vi "Test Gmail Auth.vi"() -> ()   [LabVIEW 2020]
uses:
  Gmail API/Mail Address.ctl
  Gmail API/Gmail/Gmail.lvclass
  <vilib>/IlluminatedG/IG OAuth2/OAuth2/Google/Google.lvclass
  C:/Program Files (x86)/National Instruments/LabVIEW 2020/vi.lib/IlluminatedG/IG OAuth2/OAuth2/OAuth2/OAuth2.lvclass
  <vilib>/IlluminatedG/IG OAuth2/OAuth2/OAuth2/Set Scopes.vi
  <vilib>/IlluminatedG/IG OAuth2/OAuth2/OAuth2/Launch Async Auth.vi
  Gmail API/Gmail/Add To.vi
  Gmail API/Gmail/Set Subject.vi
  Gmail API/Gmail/Set Content-Type.vi
  Gmail API/Gmail/Set Body.vi
  <vilib>/IlluminatedG/IG HTTP Utils/HTTP Utils/Response/Response.lvclass
  <vilib>/IlluminatedG/IG OAuth2/OAuth2/Authorization/Authorization.lvclass
  <vilib>/IlluminatedG/IG OAuth2/OAuth2/Client/Client.lvclass
  <vilib>/IlluminatedG/IG OAuth2/OAuth2/OAuth2/OAuth2.lvclass
  <vilib>/IlluminatedG/IG OAuth2/OAuth2/Async Authorization/Async Authorization.lvclass
  Gmail API/Gmail API.lvlib
panel:
  in  "Name":string
  in  "Content-Type":string
  in  "Body":string
  in  "Subject":string
  in  "Email":string
  in  "From Account (Prompt)":string
  in  "Secret":string
  in  "ID":string
  out "error out":errorcluster
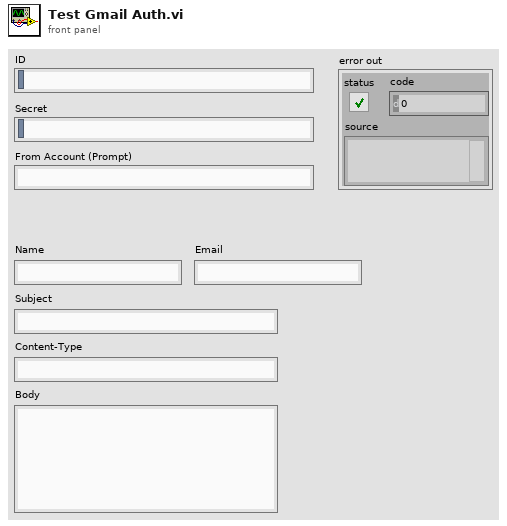
[diagram p1: front panel]
types:
  T1 = typedef "Gmail API.lvlib/Mail Address.ctl" = cluster{"Name":string, "Email":string}
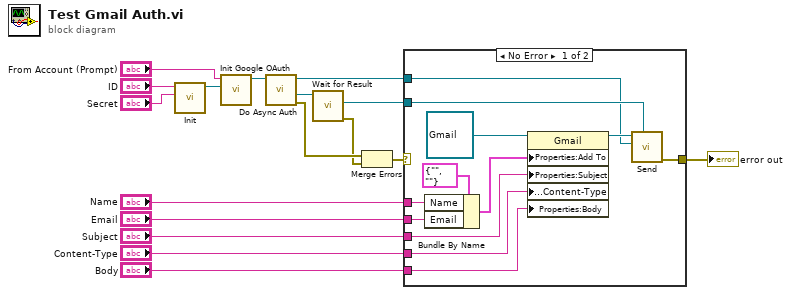
[diagram p0: block diagram]
diagram:
  n1 = call <vilib>:"Init.vi"("Secret"="Secret", "ID"="ID") -> ("Client out"=w2:refnum<class "Client.lvclass">)  [unwired: 9 in]
  n2 = call <vilib>:"Init Google OAuth.vi"("OAuth2:Client"=w2, "Account (Prompt)"="From Account (Prompt)") -> ("Google out"=w3:refnum<class "Google.lvclass">)  [unwired: 8 in, 1 out]
  n3 = call <vilib>:"Do Async Auth.vi"("OAuth2 in"=w3) -> ("error out"=w14:errorcluster, "Async Authentication"=w15:refnum<class "Async Authorization.lvclass">, "OAuth2 out"=w10:refnum<class "Google.lvclass">)  [unwired: 8 in]
  n4 = call <vilib>:"Wait for Result.vi"("Async Authorization in"=w15) -> ("error out"=w13:errorcluster, "Authorization"=w11:refnum<class "Authorization.lvclass">)  [unwired: 8 in, 1 out]
  n5 = Merge Errors(w14, w13) -> (w12:errorcluster)
  n6 = case shown="No Error" w12 {
    selector: w12 -> [_ w30]
    tunnel: w11 -> [w20 _]
    tunnel: w10 -> [w19 _]
    tunnel: "Email" -> [w27 _]
    tunnel: "Subject" -> [w25 _]
    tunnel: "Content-Type" -> [w24 _]
    tunnel: "Body" -> [w23 _]
    tunnel: "Name" -> [w28 _]
    tunnel: [w18 w30] -> w4
    frame No Error {
      n7 = Bundle By Name(cluster=T1 {"Name"="", "Email"=""} ("Mail Address"), "Name"=w28, "Email"=w27) -> (w26:T1)
      n8 = property class="Gmail"(reference=refnum<class "Gmail.lvclass"> refnum, "Properties:Add To"=w26, "Properties:Subject"=w25, "Properties:Content-Type"=w24, "Properties:Body"=w23) -> (reference out=w21:refnum<class "Gmail.lvclass">)  [unwired: 1 in, 1 out]
      n9 = call "Send.vi"("Authorization in"=w20, "Google"=w19, "Gmail in"=w21) -> ("error out"=w18:errorcluster)  [unwired: 6 in, 2 out]
    }
    frame Error {
    }
  }
  "error out" <- w4
